vi "Actor Core.vi"(8 "error in":errorcluster, 11 "Simulated User Console Actor in":refnum<class "Simulated User Console Actor.lvclass">) -> (0 "error out":errorcluster, 3 "Actor out":refnum<class "Actor.lvclass">)   [LabVIEW 2019, in "Simulated User Console Actor.lvlib" / "Simulated User Console Actor.lvclass"]
doc: "(<B>Filename</B>: Actor Framework.lvlib:Actor.lvclass:Actor Core.vi)\n\nReceives messages to the actor, reacts to them, and initiates any error handling that may shut the actor down.\n\nDescendant classes may override this VI to append parallel tasks for the actor to complete while it handles messages. Overrides use the Call Parent Method node."
uses:
  Simulated User Console Actor.lvclass
  <vilib>/ActorFramework/Actor/Actor.lvclass
  <vilib>/ActorFramework/Stop Msg/Stop Msg.lvclass
  ATM Controller/ATM Controller Messages/Set State Msg/Set State Msg.lvclass
  ATM Controller/ATM Controller/State -Enum.ctl
  ATM Controller/ATM Controller/ATM Controller.lvclass
  C:/Workspace/CLA/ATM AF/User Console Actor/User Console Actor/User Console Actor.lvclass
  C:/Program Files (x86)/National Instruments/LabVIEW 2019/vi.lib/ActorFramework/Actor/Actor.lvclass
  User Console Actor/User Console Actor/User Console Actor.lvclass
  ATM Controller/ATM Controller Messages/Press Transaction Msg/Press Transaction Msg.lvclass
  ATM Controller/ATM Controller Messages/Verfication Process Msg/Verfication Process Msg.lvclass
  ATM Controller/ATM Controller Messages/Get Account Number Msg/Set Account Number Msg.lvclass
  ATM Controller/ATM Controller Messages/Set Timeout Msg/Set Timeout Msg.lvclass
  Simulated User Console Actor Messages/Read Keypad Msg/Read Keypad Msg.lvclass
  ATM Controller/ATM Controller Messages/Withdrawal $50 Msg/Withdrawal $50 Msg.lvclass
  Keypad - Cluster.ctl
  Transactions -Cluster.ctl
panel:
  in  "Card Reader":bool
  in  "Transactions":T1
  in  "Keypad":T2
  # "[Covers: UI1]"
  # "[Covers: UI2] \n[Covers: UI2A] \n[Covers: UI2B]\n[Covers: UI2C]"
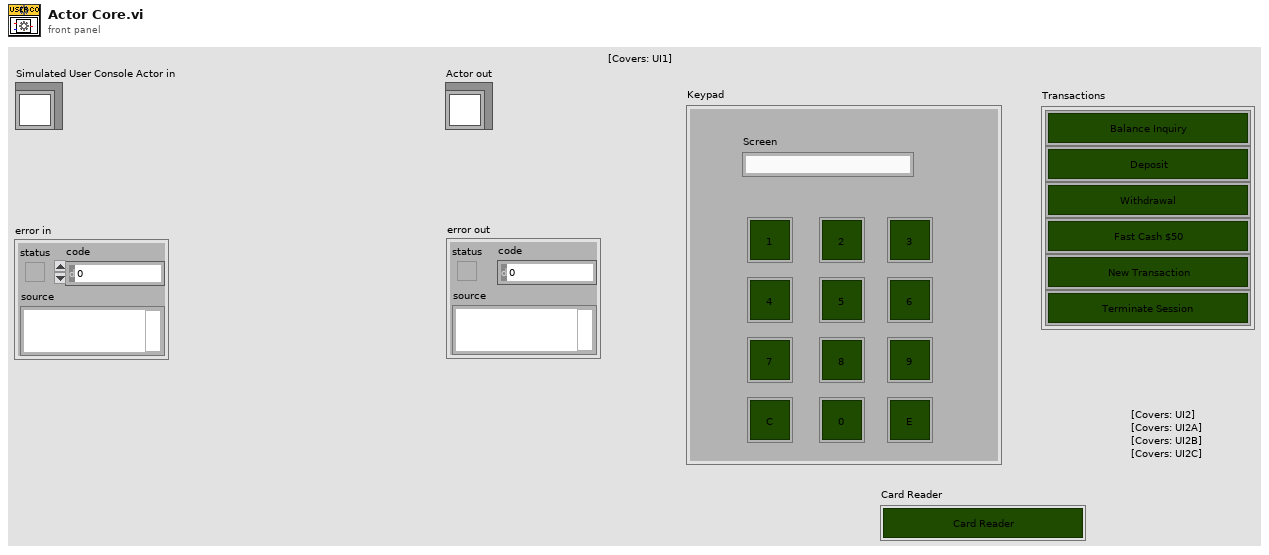
[diagram p1: front panel]
types:
  T1 = typedef "Simulated User Console Actor.lvlib/Simulated User Console Actor.lvclass/Transactions -Cluster.ctl" = cluster{"Balance Inquiry":bool, "Deposit":bool, "Withdrawal":bool, "Fast Cash $50":bool, "New Transaction":bool, "Terminate Session":bool}
  T2 = typedef "Simulated User Console Actor.lvlib/Simulated User Console Actor.lvclass/Keypad - Cluster.ctl" = cluster{"1":bool, "1 2":bool, "1 3":bool, "1 4":bool, "1 5":bool, "1 6":bool, "1 7":bool, "1 8":bool, "1 9":bool, "C":bool, "1 11":bool, "E":bool, "Screen":string}
  T3 = typedef "ATM Controller.lvlib/ATM Controller.lvclass/State -Enum.ctl" = enum16{"Inital", "Idle", "Login", "Balance Inquiry", "Deposit", "Withdrawal", "Fast Cash", "Terminate"}
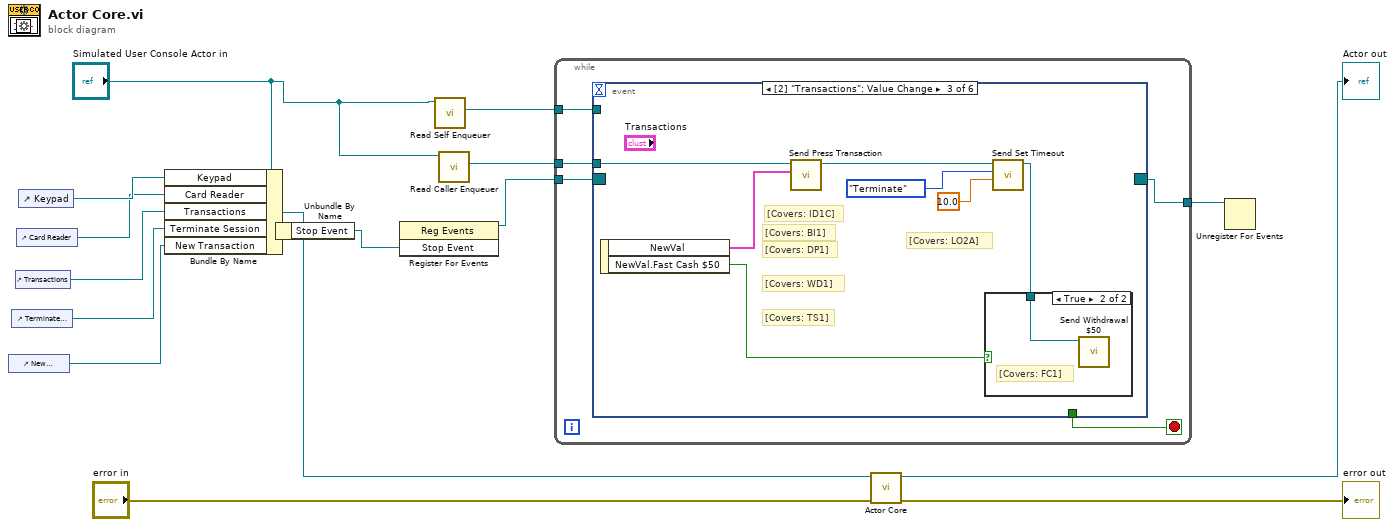
[diagram p0: block diagram]
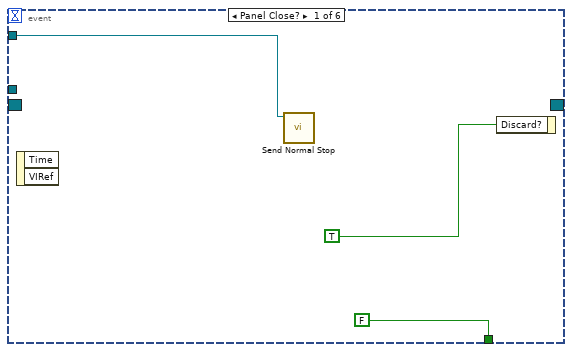
[diagram p2: hidden frame]
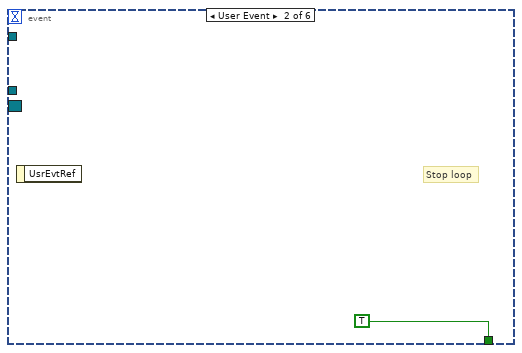
[diagram p3: hidden frame]
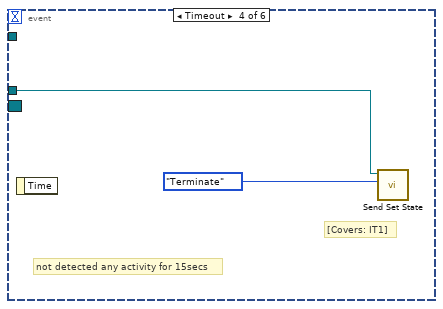
[diagram p5: hidden frame]
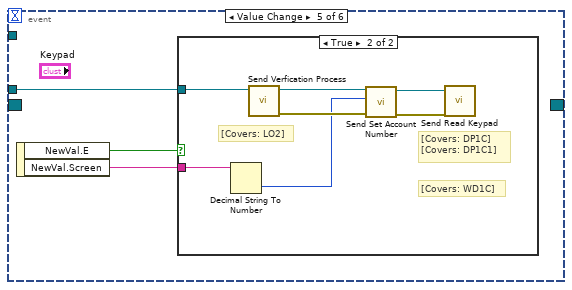
[diagram p6: hidden frame]
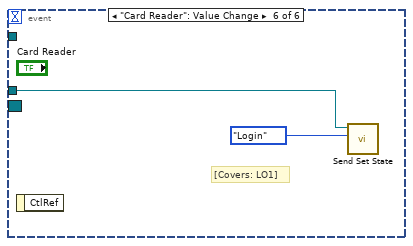
[diagram p8: hidden frame]
diagram:
  n1 = control-ref of="New Transaction"() -> (w1:refnum<vi>)
  n2 = control-ref of="Terminate Session"() -> (w2:refnum<vi>)
  n3 = control-ref of="Transactions"() -> (w5:refnum<vi>)
  n4 = control-ref of="Card Reader"() -> (w6:refnum<vi>)
  n5 = control-ref of="Keypad"() -> (w7:refnum<vi>)
  n6 = Bundle By Name(cluster="Simulated User Console Actor in", "Keypad"=w7, "Card Reader"=w6, "Transactions"=w5, "Terminate Session"=w2, "New Transaction"=w1) -> (w8:refnum<class "Simulated User Console Actor.lvclass">)
  n7 = Unbundle By Name(w8) -> ("Stop Event"=w9:refnum<user-event>)
  n8 = register-events(w9) -> (reference out=w11:refnum<event-registration>)  [unwired: 2 in, 1 out]
  n9 = call <vilib>:"Read Self Enqueuer.vi"("Actor"="Simulated User Console Actor in") -> ("Self Enqueuer"=w12:refnum<class "Message Enqueuer.lvclass">)  [unwired: 10 in]
  n10 = call <vilib>:"Read Caller Enqueuer.vi"("Actor"="Simulated User Console Actor in") -> ("Caller Enqueuer"=w4:refnum<class "Message Enqueuer.lvclass">)  [unwired: 10 in]
  n11 = while {
    tunnel: w12 -> [w19]
    tunnel: w11 -> [w18]
    tunnel: [w17] -> w10
    tunnel: w4 -> [w16]
    stop <- w20 stop-if-true
    n12 = event shown="[2] \"Transactions\": Value Change" {
      selector: w18 -> [_ _ _ _ _ _]
      dyn-events: [_ _ _ _ _ _] -> w17
      timeout: _ -> [_ _ _ _ _ _]
      tunnel: [FALSE TRUE _ _ _ _] -> w20
      tunnel: w19 -> [w22 _ _ _ _ _]
      tunnel: w16 -> [_ _ w31 w34 w37 w46]
      event Panel Close? {
        n13 = event-data() -> ()  [unwired: 1 in, 2 out]
        n14 = call <vilib>:"Send Normal Stop.vi"("Message Enqueuer"=w22) -> ()  [unwired: 10 in, 1 out]
        n15 = event-data("Discard?"=TRUE) -> ()  [unwired: 1 in, 1 out]
      }
      event User Event {
        # "Stop loop"
        n16 = event-data() -> ()  [unwired: 1 in, 1 out]
      }
      event Value Change {
        # "[Covers: LO2A]"
        # "[Covers: ID1C]"
        # "[Covers: TS1]"
        # "[Covers: WD1]"
        # "[Covers: DP1]"
        # "[Covers: BI1]"
        n17 = event-data() -> ("NewVal"=w28:T1, "NewVal.Fast Cash $50"=w26:bool)  [unwired: 1 in]
        n18 = call "Send Press Transaction.vi"("Transactions"=w28, "Message Enqueuer"=w31) -> ("Message Enqueuer out"=w30:refnum<class "Message Enqueuer.lvclass">)  [unwired: 8 in, 1 out]
        n19 = call "Send Set Timeout.vi"("Target Time"=10.0, "State"=State_-Enum."Terminate", "Message Enqueuer"=w30) -> ("Message Enqueuer out"=w25:refnum<class "Message Enqueuer.lvclass">)  [unwired: 7 in, 1 out]
        n20 = case shown="True" w26 {
          tunnel: w25 -> [_ w32]
          frame False {
          }
          frame True {
            # "[Covers: FC1]"
            n21 = call "Send Withdrawal $50.vi"("Message Enqueuer"=w32) -> ()  [unwired: 9 in, 2 out]
          }
        }
      }
      event Timeout {
        # "[Covers: IT1]"
        # "not detected any activity for 15secs"
        n22 = event-data() -> ()  [unwired: 1 in, 1 out]
        n23 = call "Send Set State.vi"("State"=State_-Enum."Terminate", "Message Enqueuer"=w34) -> ()  [unwired: 8 in, 2 out]
      }
      event Value Change {
        n24 = event-data() -> ("NewVal.E"=w36:bool, "NewVal.Screen"=w35:string)  [unwired: 1 in]
        n25 = case shown="True" w36 {
          tunnel: w37 -> [_ w44]
          tunnel: w35 -> [_ w41]
          frame False {
          }
          frame True {
            # "[Covers: WD1C]"
            # "[Covers: DP1C] \n[Covers: DP1C1]"
            # "[Covers: LO2]"
            n26 = Decimal String To Number(string=w41) -> (number=w40:i32)  [unwired: 2 in, 1 out]
            n27 = call "Send Verfication Process.vi"("Message Enqueuer"=w44) -> ("error out"=w42:errorcluster, "Message Enqueuer out"=w43:refnum<class "Message Enqueuer.lvclass">)  [unwired: 9 in]
            n28 = call "Send Set Account Number.vi"("error in (no error)"=w42, "Account Number"=w40, "Message Enqueuer"=w43) -> ("error out"=w38:errorcluster, "Message Enqueuer out"=w39:refnum<class "Message Enqueuer.lvclass">)  [unwired: 7 in]
            n29 = call "Send Read Keypad.vi"("error in (no error)"=w38, "Message Enqueuer"=w39) -> ()  [unwired: 8 in, 2 out]
          }
        }
      }
      event "Card Reader": Value Change {
        # "[Covers: LO1]"
        n30 = event-data() -> ()  [unwired: 1 in, 1 out]
        n31 = call "Send Set State.vi"("State"=State_-Enum."Login", "Message Enqueuer"=w46) -> ()  [unwired: 8 in, 2 out]
      }
    }
  }
  n32 = call-parent "Actor Core.vi"("error in"="error in", "Actor in"=w8) -> ("error out"=→"error out":errorcluster, "Actor out"=→"Actor out":refnum<class "Actor.lvclass">)  [unwired: 8 in]
  n33 = Unregister For Events(event registration refnum=w10) -> ()  [unwired: 1 in, 1 out]
